vi "Untitled 2.vi"   [LabVIEW 2024]
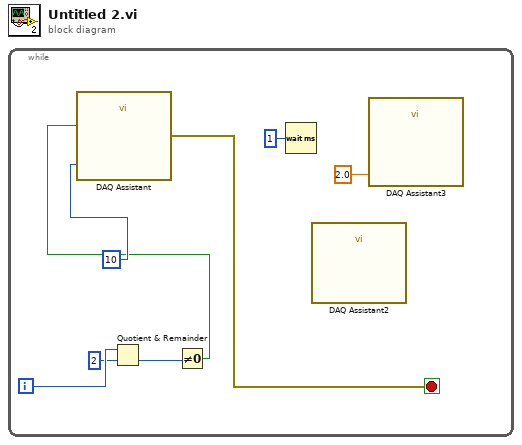
[diagram p0: block diagram]
diagram:
  n1 = while {
    i -> [w7]
    stop <- w3 stop-if-true
    n2 = Quotient & Remainder(x=w7, y=2) -> (floor(x/y)=w5:i32)  [unwired: 1 out]
    n3 = Not Equal To 0?(x=w5) -> (x != 0?=w4:bool)
    n4 = call "DAQ Assistant"("data"=10, "stop (T)"=w4) -> ("error out"=w3:errorcluster)  [unwired: 16 in, 1 out]
    n5 = Wait (ms)(milliseconds to wait=u32 1) -> ()  [unwired: 1 out]
    n6 = call "DAQ Assistant2"() -> ()  [unwired: 17 in, 3 out]
    n7 = call "DAQ Assistant3"("data"=2.0) -> ()  [unwired: 17 in, 2 out]
  }
